vi "HDF5_Init_Tone_Refs.vi"(5 "HDF5 file ref":T3 format="%.0x", 7 "ToneDataStructure":T1={"HDF5_ToneInfo"={"Timestring"="Timestamp string goes here", "Timestamp"=timestamp(0 s since 1904-01-01), "MaxValue"=0.0, "PeakLoc"=0.0, "df"=0.0}, "CalBeacArraySize"=[100000, 1], "Zoom"=array[1024 elements], "ZoomArraySize"=[100000, 1024]}, 11 "error in":errorcluster) -> (4 "ToneRefs":T4[](array[typedef]) {"Downshift_dset" format="%.0x"; "DeltaPhase_dset" format="%.0x"; "Phase_dset" format="%.0x"; "SNR_dset" format="%.0x"; "df_dset" format="%.0x"; "PeakLoc_dset" format="%.0x"; "MaxValue_dset" format="%.0x"; "TImeStamp_dset" format="%.0x"; "TimeString_dset" format="%.0x"}, 15 "error out":errorcluster)   [LabVIEW 2018]
doc: "Set up the HDF5 data structure and initialize the references for the Tone1, Tone2, Tone3, and Tone4 Groups and the datasets (tables) within each Group.\n\nData structure:\nTone1 (Group) \n Beac - cluster (Dataset)\n BeacZoom - 1024 element Double array (waveform) \n Cal - cluster\n CalZoom - 1024 element Double array (waveform) \nTone2\n Beac - cluster\n BeacZoom - 1024 element Double array (waveform) \n Cal - cluster\n CalZoom - 1024 element Double array (waveform) \nTone3\n Beac - cluster\n BeacZoom - 1024 element Double array (waveform) \n Cal - cluster\n CalZoom - 1024 element Double array (waveform) \nTone4\n Beac - cluster\n BeacZoom - 1024 element Double array (waveform) \n Cal - cluster\n CalZoom - 1024 element Double array (waveform)"
uses:
  <vilib>/addons/h5labview2/group/H5G.lvlib
  <vilib>/addons/h5labview2/dataset/H5D.lvlib
  HDF5_Tone_refs.ctl
  <vilib>/addons/h5labview2/base/hid_t.ctl
  <vilib>/addons/h5labview2/base/hid_t_renamed.ctl
  HDF5_ToneInfoClust.ctl
  ToneDataStructure.ctl
panel:
  out "Numeric":i32
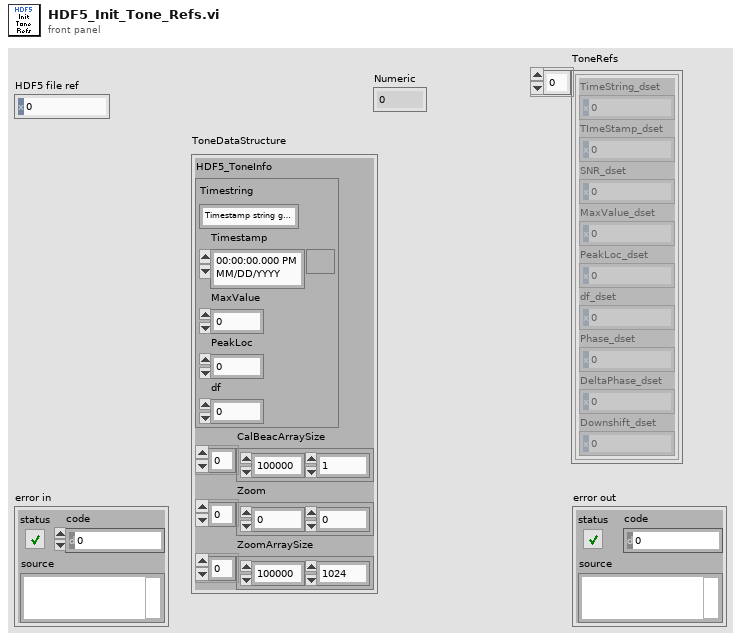
[diagram p1: front panel]
types:
  T1 = typedef "ToneDataStructure.ctl" = cluster{"HDF5_ToneInfo":T2, "CalBeacArraySize":u64[], "Zoom":dbl[], "ZoomArraySize":u64[]}
  T2 = typedef "HDF5_ToneInfoClust.ctl" = cluster{"Timestring":string, "Timestamp":timestamp, "MaxValue":dbl, "PeakLoc":dbl, "df":dbl}
  T3 = typedef "hid_t_renamed.ctl" = i32
  T4 = typedef "HDF5_Tone_refs.ctl" = cluster{"TimeString_dset":T5, "TImeStamp_dset":T5, "SNR_dset":T5, "MaxValue_dset":T5, "PeakLoc_dset":T5, "df_dset":T5, "Phase_dset":T5, "DeltaPhase_dset":T5, "Downshift_dset":T5}
  T5 = typedef "hid_t.ctl" = i32
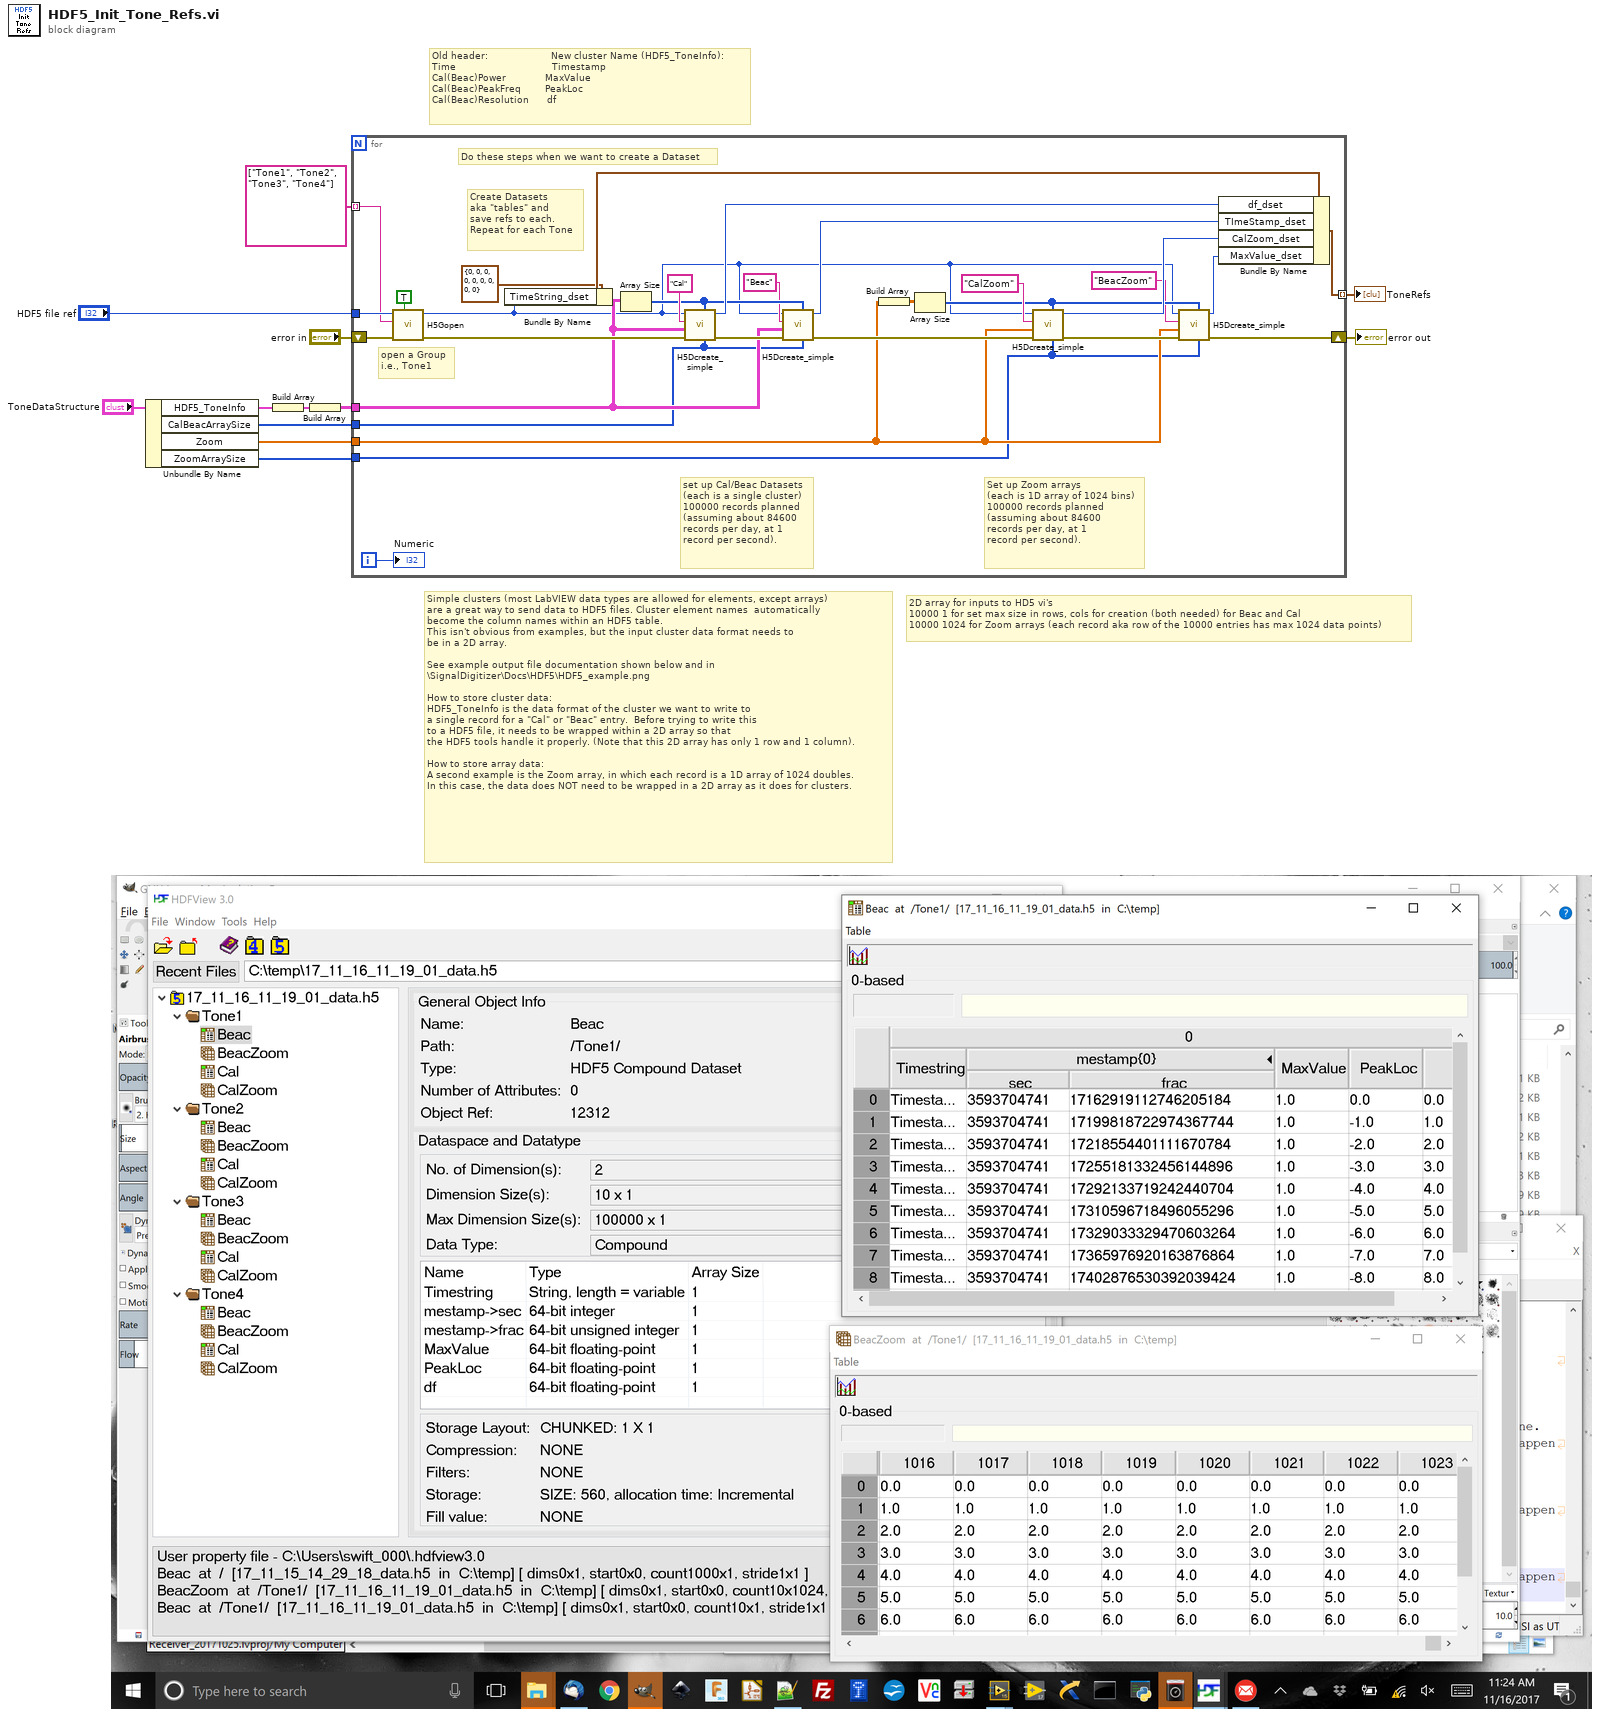
[diagram p0: block diagram]
diagram:
  # "Simple clusters (most LabVIEW data types are allowed for elements, except arrays) \nare a great way to send data to HDF5 files. Cluster element names  automatically\nbecome the column names within an HDF5 table.\nThis isn't obvious from examples, but the input cluster data format needs to \nbe in a 2D array.\n\nSee example output file documentation shown below and in\n\\SignalDigitizer\\Docs\\HDF5\\HDF5_example.png\n\nHow to store cluster data:\nHDF5_ToneInfo is the data format of the cluster we want to write to \na single record for a \"Cal\" or \"Beac\" entry.  Before trying to write this \nto a HDF5 file, it needs to be wrapped within a 2D array so that \nthe HDF5 tools handle it properly. (Note that this 2D array has only 1 row and 1 column).\n\nHow to store array data:\nA second example is the Zoom array, in which each record is a 1D array of 1024 doubles.\nIn this case, the data does NOT need to be wrapped in a 2D array as it does for clusters."
  # "2D array for inputs to HD5 vi's\n10000 1 for set max size in rows, cols for creation (both needed) for Beac and Cal\n10000 1024 for Zoom arrays (each record aka row of the 10000 entries has max 1024 data points)"
  # "Old header:                     New cluster Name (HDF5_ToneInfo):\nTime                                Timestamp\nCal(Beac)Power             MaxValue\nCal(Beac)PeakFreq        PeakLoc\nCal(Beac)Resolution      df"
  n1 = Unbundle By Name("ToneDataStructure") -> ("HDF5_ToneInfo"=w4:T2, "CalBeacArraySize"=w2:u64[], "Zoom"=w3:dbl[], "ZoomArraySize"=w1:u64[])
  n2 = Build Array(w4) -> (w9:T2[])
  n3 = Build Array(w9) -> (w8:T2[][])
  n4 = for {
    tunnel: w8 -> [w27]
    tunnel: w3 -> [w18]
    tunnel: "HDF5 file ref" -> [w41]
    shift-right: [w22] -> w6
    shift-left: "error in" -> [w38]
    tunnel: string[] ["Tone1", "Tone2", "Tone3", "Tone4"] -> [w37] mode=indexing
    tunnel: [w31] -> w12 mode=indexing
    tunnel: w2 -> [w16]
    tunnel: w1 -> [w15]
    i -> [w14]
    # "Do these steps when we want to create a Dataset"
    # "Create Datasets\naka \"tables\" and\nsave refs to each.\nRepeat for each Tone"
    # "Set up Zoom arrays\n(each is 1D array of 1024 bins)\n100000 records planned\n(assuming about 84600\nrecords per day, at 1\nrecord per second)."
    # "set up Cal/Beac Datasets\n(each is a single cluster)\n100000 records planned\n(assuming about 84600\nrecords per day, at 1\nrecord per second)."
    # "open a Group\ni.e., Tone1"
    n5 = call <vilib>:"H5Gopen.vi"("create? (F)"=TRUE, "error in (no error)"=w38, "name"=w37, "ref in"=w41) -> ("error out"=w39:errorcluster, "group out"=w20:T5)  [unwired: 6 in]
    n6 = Bundle By Name(cluster=T4 {"TimeString_dset"=0, "TImeStamp_dset"=0, "SNR_dset"=0, "MaxValue_dset"=0, "PeakLoc_dset"=0, "df_dset"=0, "Phase_dset"=0, "DeltaPhase_dset"=0, "Downshift_dset"=0} ("Cluster"), "TimeString_dset"=w20) -> (w36:T4)
    n7 = Array Size(array=w27) -> (size(s)=w29:i32[])
    n8 = call <vilib>:"H5Dcreate_simple.vi"("max size"=w16, "chunk size"=w29, "error in (no error)"=w39, "type in"=w27, "name"="Cal" ("string"), "ref in"=w20) -> ("error out"=w30:errorcluster, "dset out"=w34:T5)  [unwired: 4 in]
    n9 = call <vilib>:"H5Dcreate_simple.vi"("max size"=w16, "chunk size"=w29, "error in (no error)"=w30, "type in"=w27, "name"="Beac" ("string"), "ref in"=w20) -> ("error out"=w25:errorcluster, "dset out"=w26:T5)  [unwired: 4 in]
    n10 = Build Array(w18) -> (w35:dbl[][])
    n11 = Array Size(array=w35) -> (size(s)=w21:i32[])
    n12 = call <vilib>:"H5Dcreate_simple.vi"("max size"=w15, "chunk size"=w21, "error in (no error)"=w25, "type in"=w18, "name"="CalZoom" ("string"), "ref in"=w20) -> ("error out"=w23:errorcluster, "dset out"=w24:T5)  [unwired: 4 in]
    n13 = call <vilib>:"H5Dcreate_simple.vi"("max size"=w15, "chunk size"=w21, "error in (no error)"=w23, "type in"=w18, "name"="BeacZoom" ("string"), "ref in"=w20) -> ("error out"=w22:errorcluster, "dset out"=w17:T5)  [unwired: 4 in]
    n14 = Bundle By Name(cluster=w36, "df_dset"=w34, "TImeStamp_dset"=w26, "CalZoom_dset"=w24, "MaxValue_dset"=w17) -> (w31:T4)
    "Numeric" <- w14
  }
  "ToneRefs" <- w12
  "error out" <- w6
